vi "pump calibration dialog.vi"() -> ()   [LabVIEW 2012]
uses:
  calibration values.ctl
  calibration commands.ctl
panel:
  in  "pump ID":u8
  in  "Calculate RPM Calibration":bool
  in  "RPM Calibration":T1
  in  "STAMP Calibration":bool
  in  "STAMP intercept":dbl
  in  "STAMP slope":dbl=1.0
  in  "OK Button":bool
  in  "Set to Default":bool
  in  "Flow Calibration":T2
  in  "Save Calibration":bool
  # "scaled 0-100"
  # "scaled 0-100"
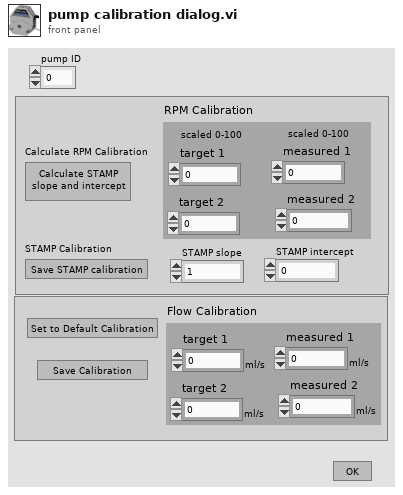
[diagram p1: front panel]
types:
  T1 = cluster{"target 1":dbl, "target 2":dbl, "measured 1":dbl, "measured 2":dbl}
  T2 = typedef "calibration values.ctl" = cluster{"target 1":dbl[unit], "target 2":dbl[unit], "measured 1":dbl[unit], "measured 2":dbl[unit]}
  T3 = typedef "calibration commands.ctl" = enum16{"Get ini Path", "Save default values", "Save new calibration", "Read calibration", "Apply calibration", "Read STAMP mb", "Write STAMP mb"}
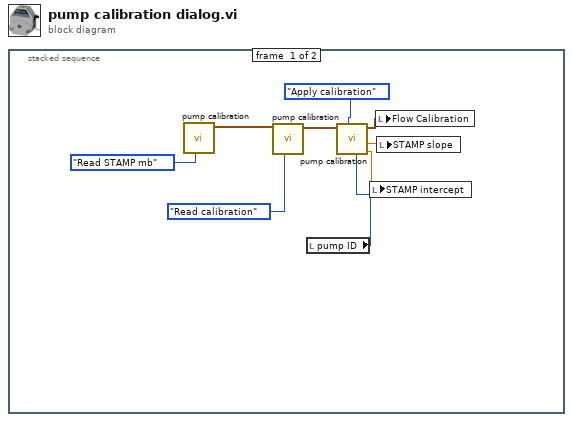
[diagram p0: block diagram]
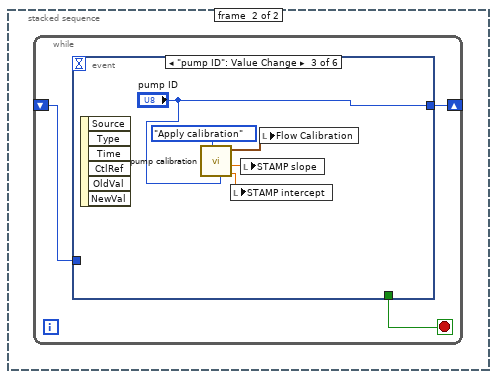
[diagram p2: hidden frame]
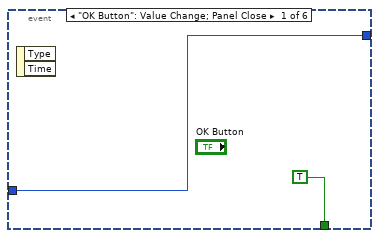
[diagram p3: hidden frame]
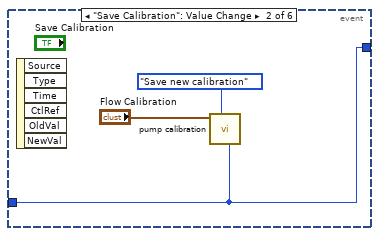
[diagram p4: hidden frame]
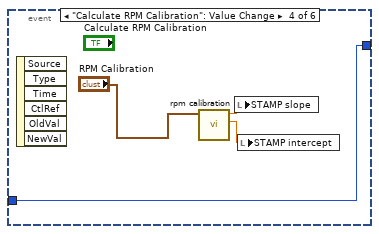
[diagram p5: hidden frame]
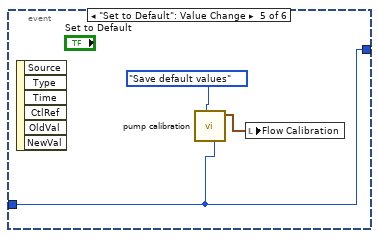
[diagram p6: hidden frame]
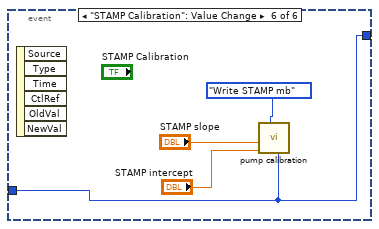
[diagram p7: hidden frame]
diagram:
  n1 = stacked-sequence {
    frame #0 {
      n2 = call "pump calibration.vi"("pump cal command"=calibration_commands."Read STAMP mb") -> ("Pump Calibration out"=w2:T2)  [unwired: 7 in, 3 out]
      n3 = call "pump calibration.vi"("pump cal command"=calibration_commands."Read calibration", "Pump Calibration in"=w2) -> ("Pump Calibration out"=w1:T2)  [unwired: 6 in, 3 out]
      n4 = local read "pump ID"() -> (w6:u8)
      n5 = call "pump calibration.vi"("pump ID"=w6, "pump cal command"=calibration_commands."Apply calibration", "Pump Calibration in"=w1) -> ("STAMP intercept out"=w9:dbl, "STAMP slope out"=w8:dbl, "Pump Calibration out"=w5:T2)  [unwired: 5 in, 1 out]
      n6 = local write "STAMP intercept"(w9) -> ()
      n7 = local write "Flow Calibration"(w5) -> ()
      n8 = local write "STAMP slope"(w8) -> ()
    }
    frame #1 {
      n9 = while {
        shift-right: [w11] -> _
        shift-left: _ -> [w10]
        stop <- w12 stop-if-true
        n10 = event shown="[2] \"pump ID\": Value Change" {
          selector: _ -> [_ _ _ _ _ _]
          dyn-events: _ -> [_ _ _ _ _ _]
          timeout: _ -> [_ _ _ _ _ _]
          tunnel: [TRUE _ _ _ _ _] -> w12
          tunnel: [w13 w15 "pump ID" w23 w27 w30] -> w11
          tunnel: w10 -> [w13 w15 _ w23 w27 w30]
          event "OK Button": Value Change; Panel Close {
            n11 = event-data() -> ()  [unwired: 1 in, 2 out]
          }
          event "Save Calibration": Value Change {
            n12 = event-data() -> ()  [unwired: 1 in, 6 out]
            n13 = call "pump calibration.vi"("pump ID"=w15, "pump cal command"=calibration_commands."Save new calibration", "Pump Calibration in"="Flow Calibration") -> ()  [unwired: 5 in, 4 out]
          }
          event "pump ID": Value Change {
            n14 = event-data() -> ()  [unwired: 1 in, 6 out]
            n15 = call "pump calibration.vi"("pump ID"="pump ID", "pump cal command"=calibration_commands."Apply calibration") -> ("STAMP intercept out"=w22:dbl, "STAMP slope out"=w21:dbl, "Pump Calibration out"=w19:T2)  [unwired: 6 in, 1 out]
            n16 = local write "STAMP intercept"(w22) -> ()
            n17 = local write "STAMP slope"(w21) -> ()
            n18 = local write "Flow Calibration"(w19) -> ()
          }
          event "Calculate RPM Calibration": Value Change {
            n19 = event-data() -> ()  [unwired: 1 in, 6 out]
            n20 = call "rpm calibration.vi"("RPM Calibration"="RPM Calibration") -> ("STAMP intercept"=w24:dbl, "STAMP slope"=w25:dbl)  [unwired: 9 in]
            n21 = local write "STAMP slope"(w25) -> ()
            n22 = local write "STAMP intercept"(w24) -> ()
          }
          event "Set to Default": Value Change {
            n23 = event-data() -> ()  [unwired: 1 in, 6 out]
            n24 = call "pump calibration.vi"("pump ID"=w27, "pump cal command"=calibration_commands."Save default values") -> ("Pump Calibration out"=w28:T2)  [unwired: 6 in, 3 out]
            n25 = local write "Flow Calibration"(w28) -> ()
          }
          event "STAMP Calibration": Value Change {
            n26 = event-data() -> ()  [unwired: 1 in, 6 out]
            n27 = call "pump calibration.vi"("pump ID"=w30, "pump cal command"=calibration_commands."Write STAMP mb", "STAMP intercept"="STAMP intercept", "STAMP slope"="STAMP slope") -> ()  [unwired: 4 in, 4 out]
          }
        }
      }
    }
  }
